vi "Get Parent Window.vi"(8 "error in":errorcluster caption="error in (no error)" {"code" format="%d\n%x"}, 11 "child window refnum":T1 caption="window refnum out") -> (0 "error out":errorcluster {"code" format="%d\n%x"}, 2 "window name":string, 3 "window refnum out":T1)   [LabVIEW 2020]
uses:
  Window Refnum.ctl
  Win Util.lvlib
  user32.dll
panel:
  in  "window name (\"\")":string
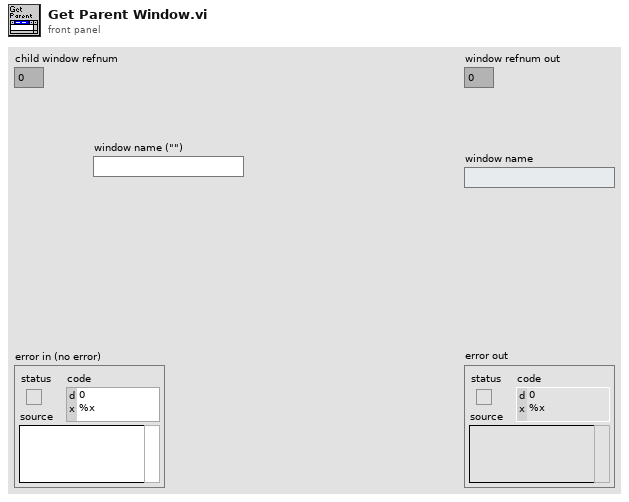
[diagram p1: front panel]
types:
  T1 = typedef "MacroAssert.lvlib/Win Util.lvlib/Window Refnum.ctl" = u64
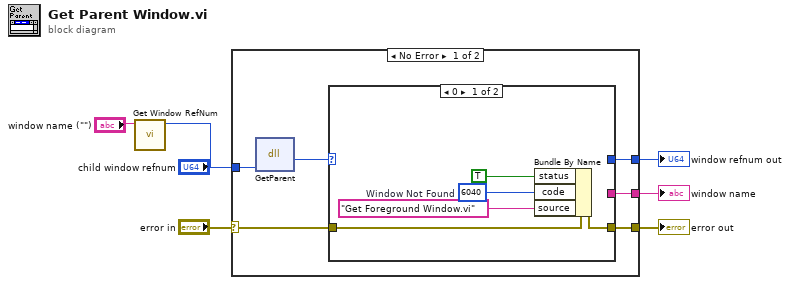
[diagram p0: block diagram]
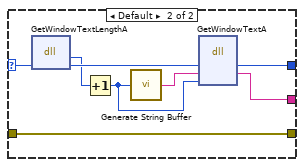
[diagram p2: hidden frame]
diagram:
  n1 = call "Get Window RefNum.vi"("window name (\"\")"="window name (\"\")") -> ("window refnum (NaWR)"=w2:T1)  [unwired: 7 in, 1 out]
  n2 = case shown="No Error" "error in" {
    selector: "error in" -> [w12 w26]
    tunnel: [w11 w26] -> w5
    tunnel: [w9 _] -> w6
    tunnel: [w8 _] -> w4
    tunnel: w2 -> [w7 _]
    frame No Error {
      n3 = dll-call lib="user32.dll" fn="GetParent"("Child hWnd"=w7) -> ("hWnd"=w10:u64)  [unwired: 3 in, 3 out]
      n4 = case shown="0" w10 {
        selector: w10 -> [_ w18]
        tunnel: w12 -> [w14 w23]
        tunnel: [w17 w23] -> w11
        tunnel: [_ w22] -> w9
        tunnel: [_ w21] -> w8
        frame 0 {
          w16 = 6040  # Window Not Found
          n5 = Bundle By Name(cluster=w14, "status"=TRUE ("show call chain? (False)"), "code"=w16, "source"="Get Foreground Window.vi") -> (w17:errorcluster)
        }
        frame Default {
          n6 = dll-call lib="user32.dll" fn="GetWindowTextLengthA" label="GetWindowTextLength"("hWnd"=w18) -> ("length"=w20:i32, "hWnd"=w24:u64)  [unwired: 3 in, 2 out]
          n7 = Increment(x=w20) -> (x+1=w19:i32)
          n8 = call "Generate String Buffer.vi"("buffer size"=w19) -> ("string buffer"=w25:string)
          n9 = dll-call lib="user32.dll" fn="GetWindowTextA" label="GetWindowText"("hWnd"=w24, "NameBuffer"=w25, "MaxCharsToCopy"=w19) -> ("hWnd"=w21:u64, "NameBuffer"=w22:string)  [unwired: 4 in, 3 out]
        }
      }
    }
    frame Error {
    }
  }
  "error out" <- w5
  "window name" <- w6
  "window refnum out" <- w4
